vi "PH_Tektronix_7000.Close.vi"(0 "i ref in":refnum<vi>, 5 "error in(no error)":errorcluster) -> (14 "i ref out":refnum<vi>, 19 "error out":errorcluster)   [LabVIEW 2014, in "PH_Tektronix_7000.lvlib"]
doc: "This VI closes the connection and sets the connection established and the error flag at own attributes to false."
uses:
  PH_Tektronix_7000.lvlib
  PH_StatusHandler/PH_StatusHandler.Status.ctl
  PH_StatusHandler/PH_StatusHandler.lvlib
  PH_Common/PH_Common.lvlib
  non_GPL/instr.lib/Tektronix 7000 Series/Tektronix 7000 Series - Driver np.lvlib
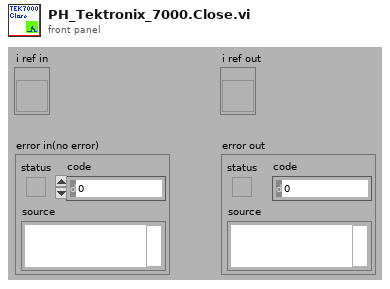
[diagram p1: front panel]
types:
  T1 = typedef "PH_Tektronix_7000.lvlib/PH_Tektronix_7000.i attribute.ctl" = cluster{"VISA Resource Name":refnum<visa-resource-name>, "IDN":cluster{"Instrument Driver":string, "Instrument Firmware":string, "Model":string, "Serial Number":string}, "Selftest":cluster{"Result":i32, "Message":string}, "Trigger Configuration":T2, "Acquisition Configuration":T3, "GUI Refs":T4, "State":T5, "Error Message":string, "Allow Prdc Loop?":bool, "Channel 1":T6, "Channel 2":T6, "Channel 3":T6, "Channel 4":T6, "Data CH 1":waveform(dbl), "Data CH 2":waveform(dbl), "Data CH 3":waveform(dbl), "Data CH 4":waveform(dbl), "Allow config?":bool, "Name Channel 1":string, "Name Channel 2":string, "Name Channel 3":string, "Name Channel 4":string, "Fetch Data before sending to PSDB?":bool, "Constructor passed?":bool, "Data taken at":timestamp, "Plot Colors":u32[], "Default VISA Resource":string}
  T2 = typedef "PH_Tektronix_7000.lvlib/PH_Tektronix_7000.Trigger Config.ctl" = cluster{"Source":u16, "Level [V]":dbl, "Slope":u16, "Coupling":u16, "Trigger Mode":u16}
  T3 = typedef "PH_Tektronix_7000.lvlib/PH_Tektronix_7000.Acquisition Config.ctl" = cluster{"Record Length":u32, "Timebase [s/div]":dbl, "Position [%]":dbl, "Acquisition Type":u16, "Average Waveforms":i32, "Envelope Waveforms":i32, "WfmDB Samples":i32, "Continuous?":bool, "Delay [s]":dbl, "Run?":bool}
  T4 = typedef "PH_Tektronix_7000.lvlib/PH_Tektronix_7000.GUI Refs.ctl" = cluster{"Graph":refnum<vi>, "State":refnum<vi>, "Delete":refnum<vi>, "VISA Resource":refnum<vi>, "Allow Configure":refnum<vi>, "Fetch Data":refnum<vi>, "Fetch before sending Data to PSDB":refnum<vi>, "Name Channel 1":refnum<vi>, "Name Channel 2":refnum<vi>, "Name Channel 3":refnum<vi>, "Name Channel 4":refnum<vi>, "Prdc Intervall [ms]":refnum<vi>, "Data taken":refnum<vi>, "Model":refnum<vi>, "Serial Number":refnum<vi>, "Firmware":refnum<vi>, "Driver":refnum<vi>, "Acquisition":refnum<vi>, "Trigger":refnum<vi>, "Cursor: D Time [s]":refnum<vi>, "Cursor: D Signal [V]":refnum<vi>, "Channel 1":refnum<vi>, "Channel 2":refnum<vi>, "Channel 3":refnum<vi>, "Channel 4":refnum<vi>}
  T5 = typedef "PH_StatusHandler.lvlib/PH_StatusHandler.Status.ctl" = i16
  T6 = typedef "PH_Tektronix_7000.lvlib/PH_Tektronix_7000.Channel Config.ctl" = cluster{"Enable Channel":bool, "Bandwidth":u16, "Input Impedance":u16, "Vertical Coupling":u16, "Probe Attenuation":dbl, "Range [V/div]":dbl, "Position [div]":dbl, "Bandwidth raw":string}
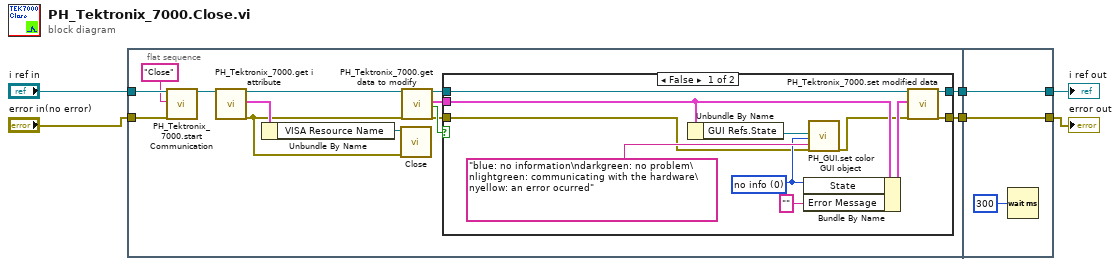
[diagram p0: block diagram]
diagram:
  n1 = flat-sequence {
    tunnel: "error in(no error)" -> [w19]
    tunnel: "i ref in" -> [w9]
    tunnel: [w16] -> w2
    tunnel: [w15] -> w1
    tunnel: [w35] -> w4
    tunnel: [w36] -> w5
    tunnel: w2 -> [w36]
    tunnel: w1 -> [w35]
    frame #0 {
      n2 = call "PH_Tektronix_7000.start Communication.vi"("i ref in"=w9, "Action"="Close", "error in"=w19) -> ("i ref out"=w7:refnum<vi>)  [unwired: 15 in, 1 out]
      n3 = call "PH_Tektronix_7000.get i attribute.vi"("i ref in"=w7) -> ("i ref out"=w17:refnum<vi>, "i attribute"=w20:T1, "error out"=w10:errorcluster)  [unwired: 16 in]
      n4 = Unbundle By Name(w20) -> ("VISA Resource Name"=w11:refnum<visa-resource-name>)
      n5 = call "Close.vi"("error in (no error)"=w10, "VISA resource name"=w11) -> ()  [unwired: 9 in, 1 out]
      n6 = call "PH_Tektronix_7000.get data to modify.vi"("i ref in"=w17, "error in (no error)"=w10) -> ("i ref out"=w14:refnum<vi>, "i attribute"=w13:T1, "timed out"=w18:bool, "error out"=w12:errorcluster)  [unwired: 14 in]
      n7 = case shown="False" w18 {
        tunnel: [w31 w32] -> w15
        tunnel: w12 -> [w22 w32]
        tunnel: w14 -> [w30 w33]
        tunnel: [w29 w33] -> w16
        tunnel: w13 -> [w26 _]
        frame False {
          w23 = T5 0 items=["no info", "off/false/out", "on/true/in", "Failure", "Alarm", "Status 1", "Status 2", "Status 3"] ("State")
          n8 = Unbundle By Name(w26) -> ("GUI Refs.State"=w25:refnum<vi>)
          n9 = Bundle By Name(cluster=w26, "State"=w23, "Error Message"="" ("Error.Message")) -> (w28:T1)
          n10 = call "PH_GUI.set color GUI object.vi"("GUI object Ref"=w25, "State"=w23, "error in (no error)"=w22, "Tip Strip (N/A)"="blue: no information\ndarkgreen: no problem\nlightgreen: communicating with the hardware\nyellow: an error ocurred") -> ("error out"=w21:errorcluster)  [unwired: 15 in]
          n11 = call "PH_Tektronix_7000.set modified data.vi"("i ref in"=w30, "i attribute"=w28, "error in (no error)"=w21) -> ("i ref out"=w29:refnum<vi>, "error out"=w31:errorcluster)  [unwired: 15 in]
        }
        frame True {
        }
      }
    }
    frame #1 {
      n12 = Wait (ms)(milliseconds to wait=u32 300) -> ()  [unwired: 1 out]
    }
  }
  "error out" <- w4
  "i ref out" <- w5
